vi "Raw2ProperNaming(SubVI).vi"(7 "AE-NamesMapping":T3(array[cluster]), 11 "Report Data":T1) -> (3 "Report Data out":T1)   [LabVIEW 2017, in "DS_Lib.lvlib" / "SRReportParser.lvlib"]
uses:
  SRReportParser.lvlib
  Modules/Private Controls/Report Data Cluster.ctl
  Modules/Private Controls/Data Raw.ctl
  Modules/Data Operations.lvlib
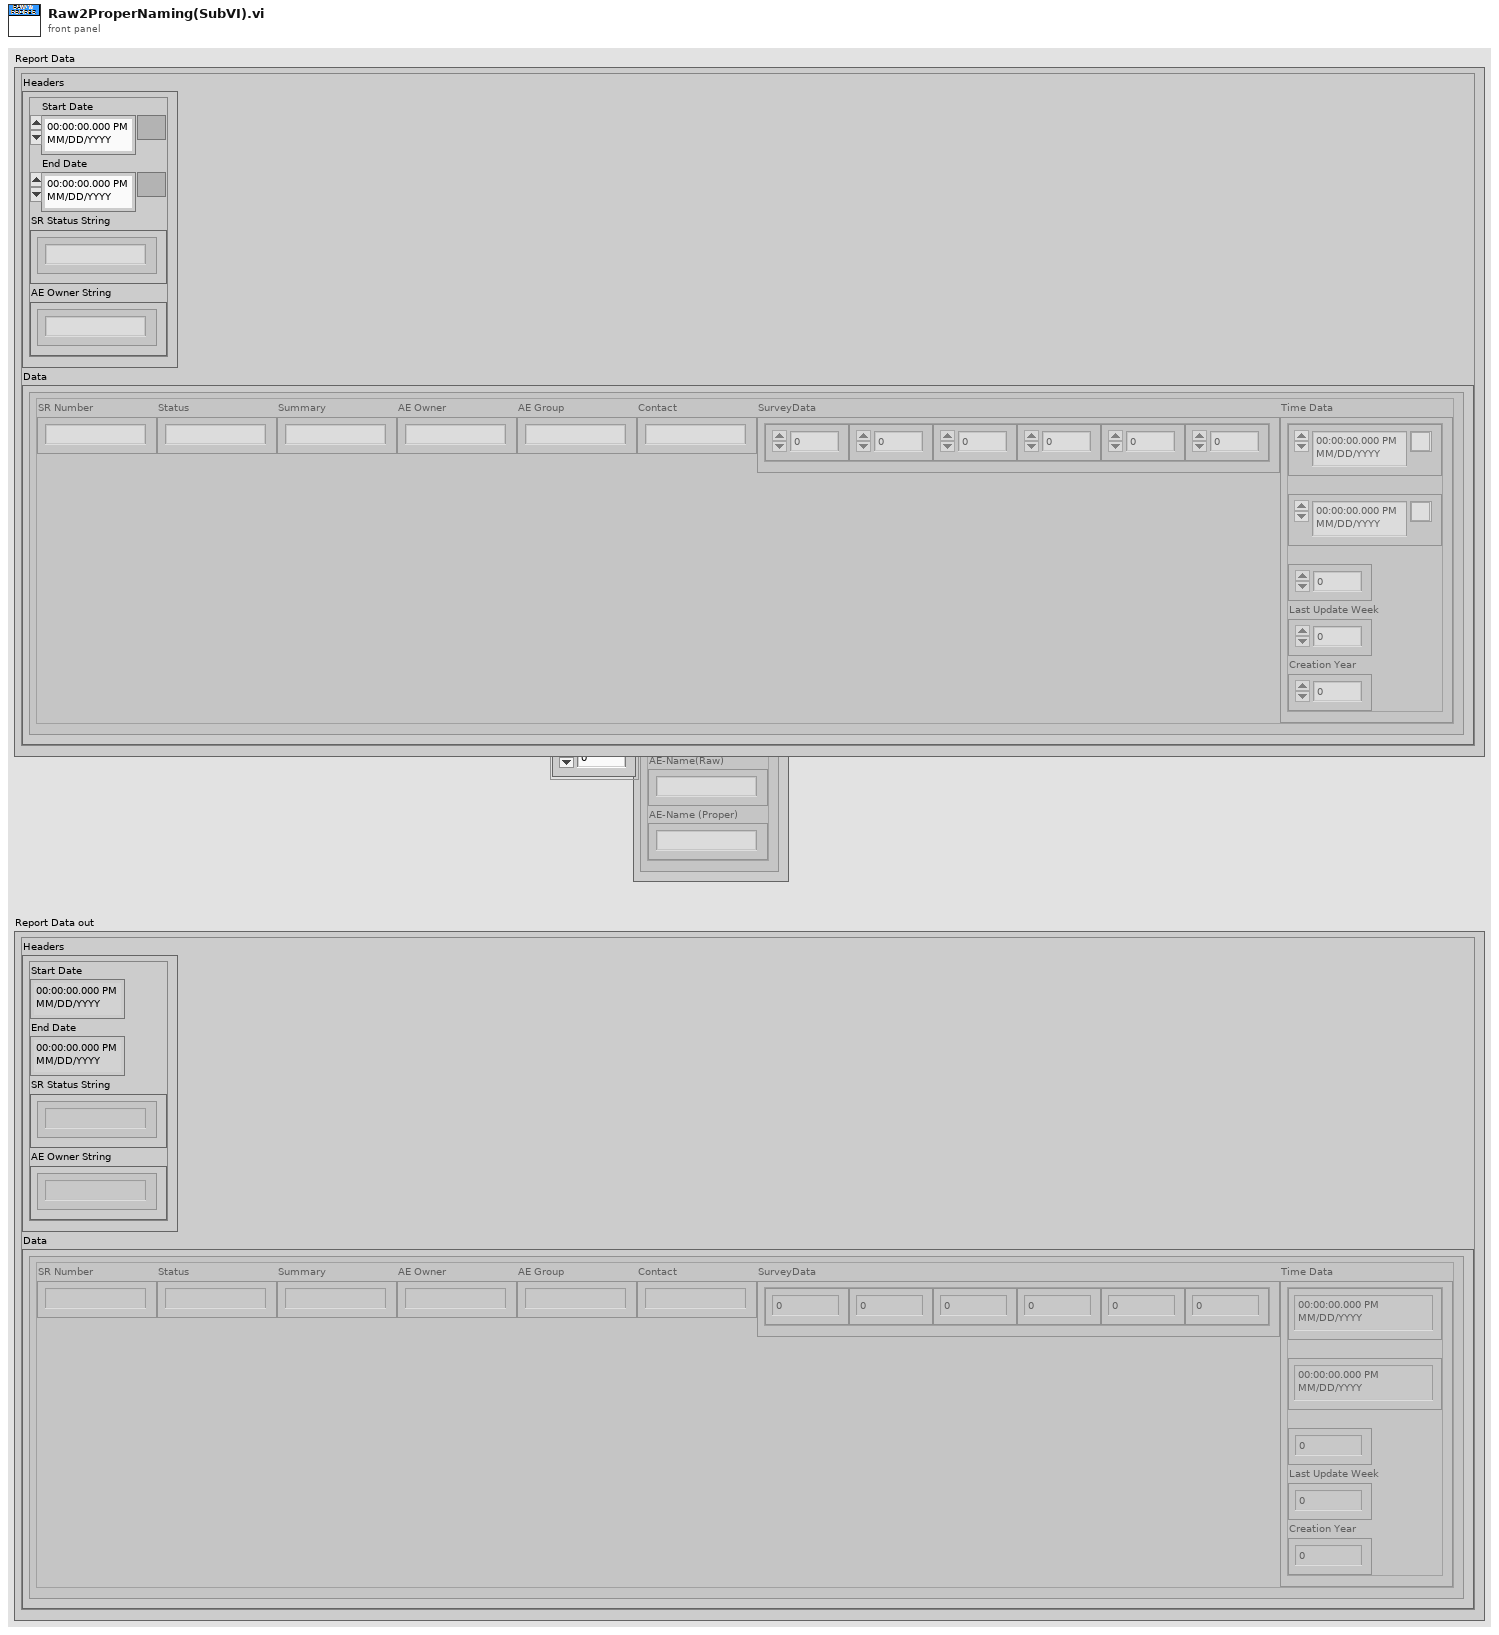
[diagram p1: front panel]
types:
  T1 = typedef "Data Operations.lvlib/Report Data Cluster.ctl" = cluster{"Headers":cluster{"Start Date":timestamp, "End Date":timestamp, "SR Status String":string[], "AE Owner String":string[]}, "Data":T2[]}
  T2 = typedef "Data Operations.lvlib/Data Raw.ctl" = cluster{"SR Number":string, "Status":string, "Summary":string, "AE Owner":string, "AE Group":string, "Contact":string, "SurveyData":cluster{"Resolution Time":dbl, "Total Satisfaction":dbl, "Response Time":dbl, "Courtesy":dbl, "Problem Solved":dbl, "Level of effort":dbl}, "Time Data":cluster{"Last Update Date":timestamp, "Creation Date":timestamp, "Creation week":i16, "Last Update Week":i16, "Creation Year":i16}}
  T3 = cluster{"AE-Name(Raw)":string, "AE-Name (Proper)":string}[]
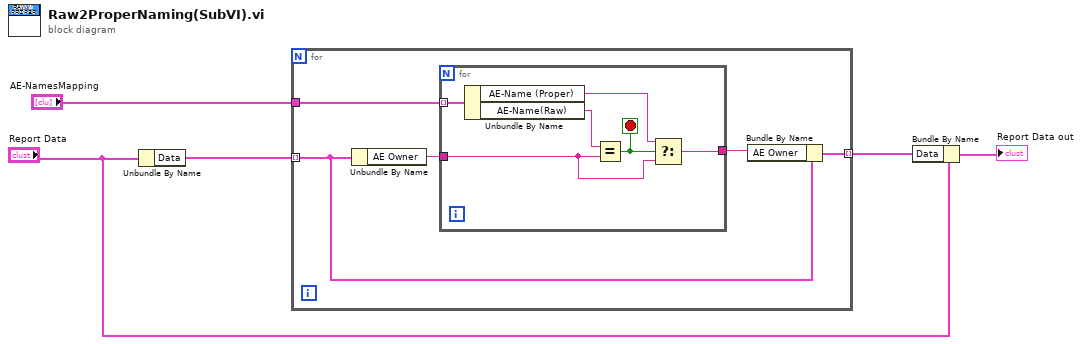
[diagram p0: block diagram]
diagram:
  n1 = Unbundle By Name("Report Data") -> ("Data"=w4:T2[])
  n2 = for {
    tunnel: w4 -> [w8] mode=indexing
    tunnel: "AE-NamesMapping" -> [w9]
    tunnel: [w6] -> w3 mode=indexing
    n3 = Unbundle By Name(w8) -> ("AE Owner"=w10:string)
    n4 = for {
      tunnel: w10 -> [w13]
      tunnel: w9 -> [w16] mode=indexing
      tunnel: [w12] -> w7
      stop <- w11 stop-if-true
      n5 = Unbundle By Name(w16) -> ("AE-Name (Proper)"=w14:string, "AE-Name(Raw)"=w15:string)
      n6 = Equal?(x=w15, y=w13) -> (x = y?=w11:bool)
      n7 = Select(t=w14, s=w11, f=w13) -> (s? t:f=w12:string)
    }
    n8 = Bundle By Name(cluster=w8, "AE Owner"=w7) -> (w6:T2)
  }
  n9 = Bundle By Name(cluster="Report Data", "Data"=w3) -> (→"Report Data out":T1)
